vi "Do This.vi"(8 "error in (no error)":errorcluster, 10 "Status Events":refnum<class "Status Events.lvclass">, 11 "VIPB Build in":refnum<class "VIPB Build.lvclass">) -> (0 "error out":errorcluster, 3 "VIPB Build out":refnum<class "VIPB Build.lvclass">)   [LabVIEW 2014, in "VIPB Build.lvclass"]
uses:
  VIPB Build.lvclass
  Shared/Classes/Status Events/Status Events.lvclass
  Classes/Job/Job.lvclass/Job.ctl
  VIPB Build.lvclass/VIPB Build.ctl
  <vilib>/Utility/error.llb/DialogType.ctl
  <vilib>/JKI/VIPM API/VIPM API_vipm_api.lvlib
  Classes/Job/Job.lvclass
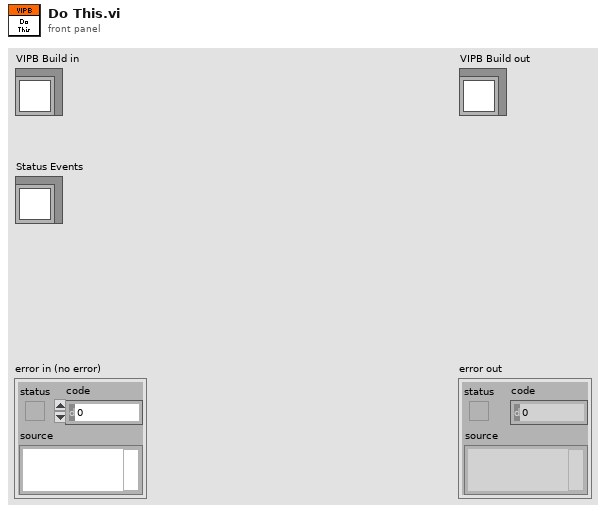
[diagram p1: front panel]
types:
  T1 = typedef "DialogType.ctl" = u16
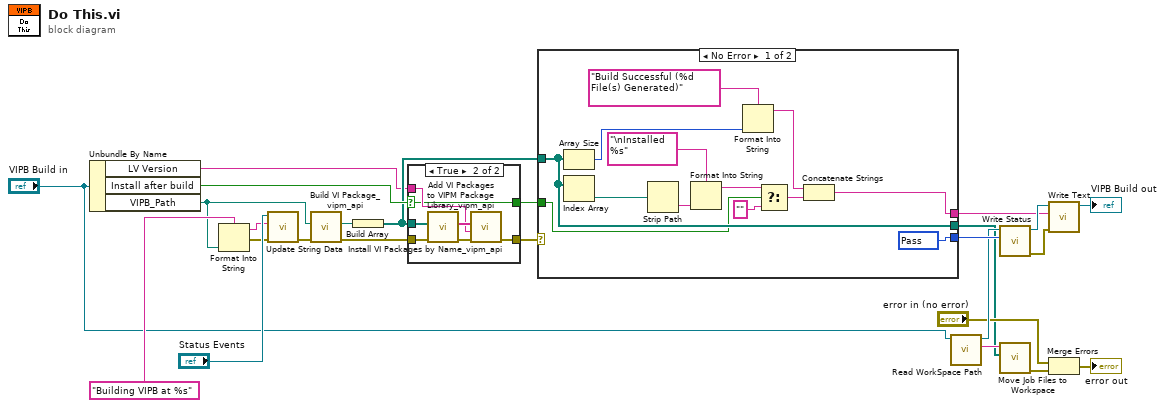
[diagram p0: block diagram]
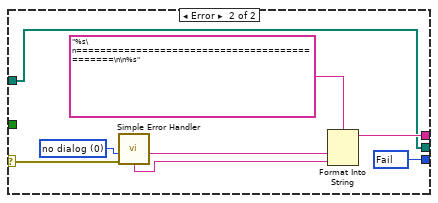
[diagram p3: hidden frame]
diagram:
  n1 = Unbundle By Name("VIPB Build in") -> ("LV Version"=w2:string, "Install after build"=w5:bool, "VIPB_Path"=w7:path)
  n2 = Format Into String(format string="Building VIPB at %s", w7) -> (resulting string=w24:string, error out=w9:errorcluster)  [unwired: 2 in]
  n3 = call "Update String Data.vi"("error in (no error)"=w9, "String Data"=w24, "Status Updater in"="Status Events") -> ("error out"=w8:errorcluster)  [unwired: 7 in, 1 out]
  n4 = call <vilib>:"Build VI Package_vipm_api.vi"("error in (no error)"=w8, "Path to VIPB File"=w7) -> ("error out"=w6:errorcluster, "Build Output"=w20:path)  [unwired: 8 in]
  n5 = Build Array(w20) -> (w4:path[])
  n6 = case shown="True" w5 {
    selector: w5 -> [w26 w28]
    tunnel: [w27 w32] -> w3
    tunnel: w6 -> [w27 w31]
    tunnel: w4 -> [_ w30]
    tunnel: w2 -> [_ w29]
    tunnel: [w26 w28] -> w1
    frame False {
    }
    frame True {
      n7 = call <vilib>:"Add VI Packages to VIPM Package Library_vipm_api.vi"("error in (no error)"=w31, "Packages to add to VIPM Library (vipc,vip,ogp)"=w30) -> ("error out"=w34:errorcluster, "Package Names Added"=w33:string[])  [unwired: 8 in]
      n8 = call <vilib>:"Install VI Packages by Name_vipm_api.vi"("error in (no error)"=w34, "LabVIEW Version"=w29, "Package Names to Install []"=w33) -> ("error out"=w32:errorcluster)  [unwired: 8 in]
    }
  }
  n9 = case shown="No Error" w3 {
    selector: w3 -> [_ w54]
    tunnel: [w47 w55] -> w16
    tunnel: [w35 w49] -> w17
    tunnel: w4 -> [w42 w48]
    tunnel: [w42 w48] -> w10
    tunnel: w1 -> [w37 _]
    frame No Error {
      w47 = u16 200 items=["Abort"=503, "Fail"=500, "Pass"=200] ("Status")
      n10 = Array Size(array=w42) -> (size(s)=w45:i32)
      n11 = Index Array(array=w42) -> (element=w41:path)  [unwired: 1 in]
      n12 = Strip Path(path=w41) -> (name=w43:string)  [unwired: 1 out]
      n13 = Format Into String(format string="\nInstalled %s", w43) -> (resulting string=w38:string)  [unwired: 2 in, 1 out]
      n14 = Format Into String(format string="Build Successful (%d File(s) Generated)" ("Text"), w45) -> (resulting string=w40:string)  [unwired: 2 in, 1 out]
      n15 = Select(t=w38, s=w37, f="") -> (s? t:f=w39:string)
      n16 = Concatenate Strings(w40, w39) -> (w35:string)
    }
    frame Error {
      w53 = T1 0 items=["no dialog", "OK message", "continue or stop message", "OK message + warnings", "continue/stop + warnings"] ("type of dialog (OK msg:1)")
      w55 = u16 500 items=["Abort"=503, "Fail"=500, "Pass"=200] ("Status")
      n17 = call <vilib>:"Simple Error Handler.vi"("type of dialog (OK msg:1)"=w53, "error in (no error)"=w54) -> ("source out"=w51:string, "message"=w50:string)  [unwired: 3 in, 3 out]
      n18 = Format Into String(format string="%s\n==============================================\n\n%s", w51, w50) -> (resulting string=w49:string)  [unwired: 2 in, 1 out]
    }
  }
  n19 = call "Read WorkSpace Path.vi"("Job in"="VIPB Build in") -> ("WorkSpace Path"=w21:string, "Job out"=w15:refnum<class "VIPB Build.lvclass">)  [unwired: 8 in, 1 out]
  n20 = call "Write Status.vi"("Status"=w16, "Job in"=w15) -> ("error out"=w18:errorcluster, "Job out"=w19:refnum<class "VIPB Build.lvclass">)  [unwired: 8 in]
  n21 = call "Move Job Files to Workspace.vi"("Generated Files"=w10, "Workspace Path"=w21) -> ("error out"=w11:errorcluster)  [unwired: 9 in]
  n22 = call "Write Text.vi"("error in (no error)"=w18, "Text"=w17, "Job in"=w19) -> ("Job out"=→"VIPB Build out":refnum<class "VIPB Build.lvclass">)  [unwired: 7 in, 1 out]
  n23 = Merge Errors("error in (no error)", w11) -> (→"error out":errorcluster)
